vi "extract_basic_log.vi"(9 "Next element index":i32, 10 "Current element index":i32, 11 "total string":string) -> (3 "Cluster of named data":T1 {"SailPositions"."MainSailSuggestion" min=0.0 max=1.0; "SailPositions"."JibSailSuggestion" min=0.0 max=1.0; "RudderPosition" min=-0.95 max=0.95 scale=1.0..-1.0; "BoatLocation"."North" format="%#_10f"; "BoatLocation"."East" format="%#_8f"})   [LabVIEW 2013]
doc: "Extracts the data from a basic log message, as saved by write_basic_log. If the data types saved are different from those extracted there wll be problems.\n\nEric Schneider, October 2014"
uses:
  Data/TypeDefs/BasicLogging.ctl
  Data/TypeDefs/BasicLogReading.ctl
  Data/TypeDefs/Sail Set Suggestions.ctl
  Data/TypeDefs/Rudder Set Suggestions.ctl
  Data/TypeDefs/UTM Location.ctl
panel:
  out "Extracted array":T5[](array[typedef])
  out "Data substring":string
  out "Single message substring":string
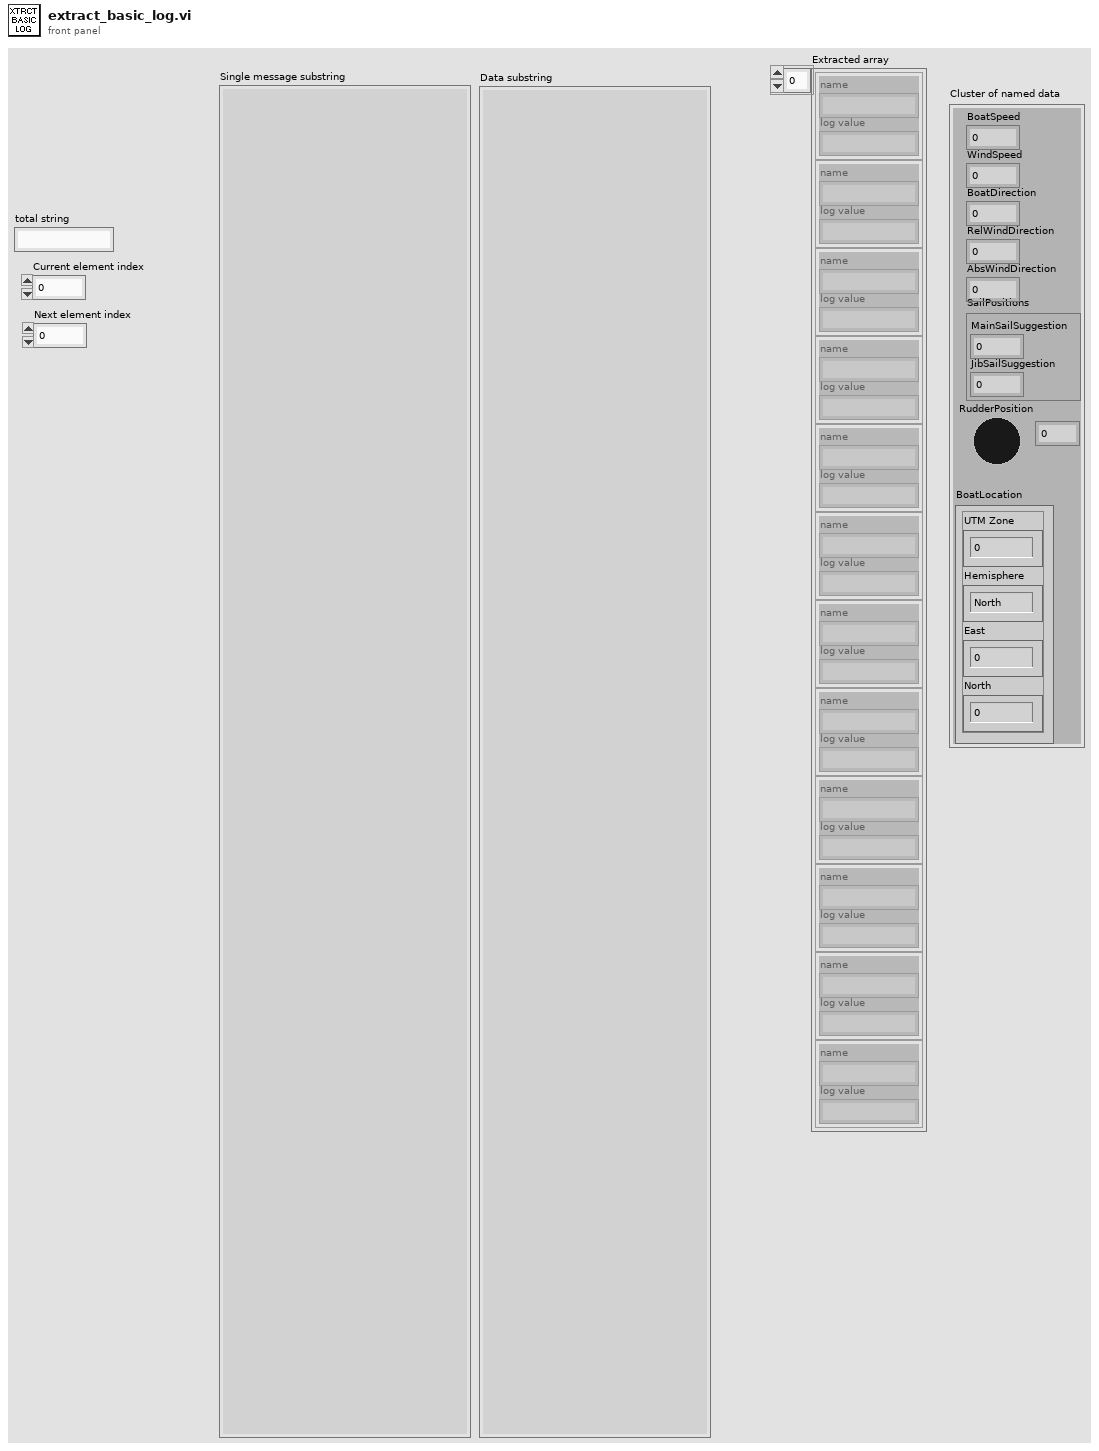
[diagram p1: front panel]
types:
  T1 = typedef "BasicLogReading.ctl" = cluster{"BoatSpeed":dbl, "WindSpeed":dbl, "BoatDirection":dbl, "RelWindDirection":dbl, "AbsWindDirection":dbl, "SailPositions":T2, "RudderPosition":T3, "BoatLocation":T4}
  T2 = typedef "Sail Set Suggestions.ctl" = cluster{"MainSailSuggestion":dbl, "JibSailSuggestion":dbl}
  T3 = typedef "Rudder Set Suggestions.ctl" = dbl
  T4 = typedef "UTM Location.ctl" = cluster{"UTM Zone":dbl, "Hemisphere":enum16{"North", "South"}, "East":dbl, "North":dbl}
  T5 = typedef "BasicLogging.ctl" = cluster{"name":string, "log value":string}
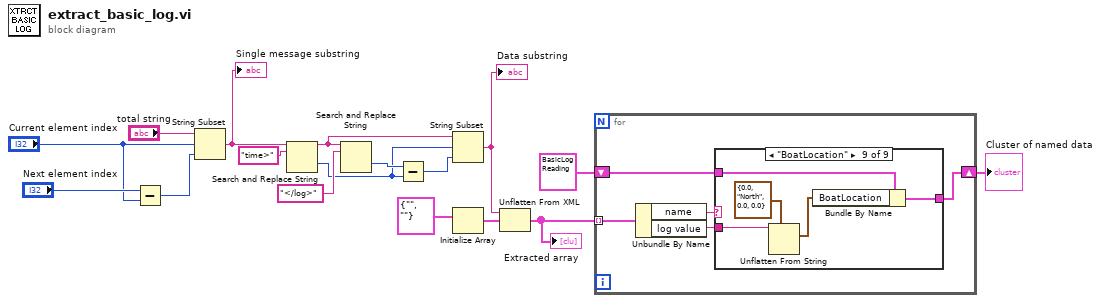
[diagram p0: block diagram]
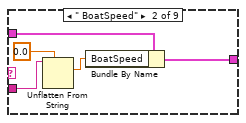
[diagram p3: hidden frame]
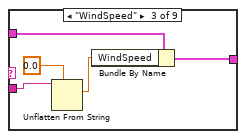
[diagram p4: hidden frame]
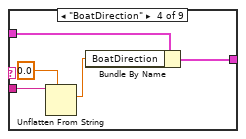
[diagram p5: hidden frame]
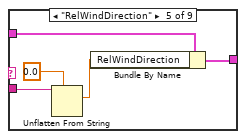
[diagram p6: hidden frame]
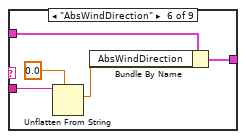
[diagram p7: hidden frame]
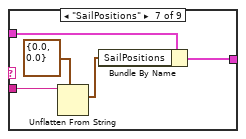
[diagram p8: hidden frame]
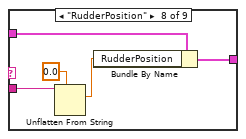
[diagram p9: hidden frame]
diagram:
  n1 = Subtract(x="Next element index", y="Current element index") -> (x-y=w16:i32)
  n2 = String Subset(string="total string", offset (0)="Current element index", length (rest)=w16) -> (substring=w13:string)
  "Single message substring" <- w13
  n3 = Search and Replace String(input string=w13, search string="time>") -> (result string=w11:string, offset past replacement=w8:i32)  [unwired: 6 in, 2 out]
  n4 = Search and Replace String(input string=w11, search string="</log>") -> (offset past replacement=w9:i32)  [unwired: 6 in, 3 out]
  n5 = Subtract(x=w9, y=w8) -> (x-y=w7:i32)
  n6 = String Subset(string=w11, offset (0)=w8, length (rest)=w7) -> (substring=w6:string)
  "Data substring" <- w6
  n7 = Initialize Array(T5 {"name"="", "log value"=""}) -> (w4:T5[])  [unwired: 1 in]
  n8 = Unflatten From XML(xml string=w6, type=w4) -> (value=w3:T5[])  [unwired: 1 in, 1 out]
  "Extracted array" <- w3
  n9 = for {
    tunnel: w3 -> [w22] mode=indexing
    shift-right: [w19] -> w1
    shift-left: T1 {"BoatSpeed"=0.0, "WindSpeed"=0.0, "BoatDirection"=0.0, "RelWindDirection"=0.0, "AbsWindDirection"=0.0, "SailPositions"={"MainSailSuggestion"=0.0, "JibSailSuggestion"=0.0}, "RudderPosition"=0.0, "BoatLocation"={"UTM Zone"=0.0, "Hemisphere"=enum."North", "East"=0.0, "North"=0.0}} -> [w18]
    n10 = Unbundle By Name(w22) -> ("name"=w21:string, "log value"=w20:string)
    n11 = case shown="\"BoatLocation\"" w21 {
      tunnel: w20 -> [_ w26 w32 w36 w42 w46 w50 w56 w62]
      tunnel: w18 -> [w23 w27 w31 w35 w40 w45 w52 w55 w61]
      tunnel: [w23 w28 w30 w34 w39 w44 w49 w54 w60] -> w19
      frame Default {
      }
      frame " BoatSpeed" {
        n12 = Unflatten From String(type=0.0 ("BoatSpeed"), binary string=w26) -> (value=w24:dbl)  [unwired: 3 in, 2 out]
        n13 = Bundle By Name(cluster=w27, "BoatSpeed"=w24) -> (w28:T1)
      }
      frame "WindSpeed" {
        n14 = Unflatten From String(type=0.0 ("x+y"), binary string=w32) -> (value=w29:dbl)  [unwired: 3 in, 2 out]
        n15 = Bundle By Name(cluster=w31, "WindSpeed"=w29) -> (w30:T1)
      }
      frame "BoatDirection" {
        n16 = Unflatten From String(type=0.0 ("x+y"), binary string=w36) -> (value=w37:dbl)  [unwired: 3 in, 2 out]
        n17 = Bundle By Name(cluster=w35, "BoatDirection"=w37) -> (w34:T1)
      }
      frame "RelWindDirection" {
        n18 = Unflatten From String(type=0.0 ("x+y"), binary string=w42) -> (value=w41:dbl)  [unwired: 3 in, 2 out]
        n19 = Bundle By Name(cluster=w40, "RelWindDirection"=w41) -> (w39:T1)
      }
      frame "AbsWindDirection" {
        n20 = Unflatten From String(type=0.0 ("x+y"), binary string=w46) -> (value=w47:dbl)  [unwired: 3 in, 2 out]
        n21 = Bundle By Name(cluster=w45, "AbsWindDirection"=w47) -> (w44:T1)
      }
      frame "SailPositions" {
        n22 = Unflatten From String(type=T2 {"MainSailSuggestion"=0.0, "JibSailSuggestion"=0.0} ("latest notification"), binary string=w50) -> (value=w53:T2)  [unwired: 3 in, 2 out]
        n23 = Bundle By Name(cluster=w52, "SailPositions"=w53) -> (w49:T1)
      }
      frame "RudderPosition" {
        n24 = Unflatten From String(type=T3 0.0 ("latest notification"), binary string=w56) -> (value=w57:T3)  [unwired: 3 in, 2 out]
        n25 = Bundle By Name(cluster=w55, "RudderPosition"=w57) -> (w54:T1)
      }
      frame "BoatLocation" {
        n26 = Unflatten From String(type=T4 {"UTM Zone"=0.0, "Hemisphere"=enum."North", "East"=0.0, "North"=0.0} ("latest notification"), binary string=w62) -> (value=w63:T4)  [unwired: 3 in, 2 out]
        n27 = Bundle By Name(cluster=w61, "BoatLocation"=w63) -> (w60:T1)
      }
    }
  }
  "Cluster of named data" <- w1
